vi "Wait for Stream.vi"(5 "timeout in milliseconds":u32=5000, 8 "error in (no error)":errorcluster, 9 "wait for samples transferred":i64=-1, 10 "stream index":i32, 11 "refnum in":refnum<k20>) -> (0 "error out":errorcluster, 1 "samples transferred":u64, 2 "stream state":T1, 3 "refnum out":refnum<k20>)   [LabVIEW 2015, in "niInstr Streaming v1 Host.lvlib"]
doc: "Wait for the specified stream to enter a terminal state (any state that is not Finite or Continuous), or for it to transfer the specified number of samples. If it does not before the timeout is reached, then the VI will throw a timeout error.\n\nSpecifying -1 (the default) for <b>wait for samples transferred</b> shall cause the VI to ignore the number of samples transferred, and only exit on the stream stopping or a timeout.\n\nSpecifying 0 for <b>wait for samples transferred</b> shall cause the VI to immediately return, regardless as to samples transferred. The current number of samples transferred will be reported, as will the stream state.\n\nSpecifying any positive number for <b>wait for samples transferred</b> shall cause the VI to block until that number of samples is reported as transferred, or until the timeout is reached.\n\nThe number of samples transferred is queried after the state, so if the <B>stream state</B> reports \"Done\" - then the samples transferred accurately reflects the terminal state of the stream. However, it is possible for the stream to report that it is still active, but have the number of samples transferred that would indicate completion.\n\nIf the stream enters the Error state, this VI will immediately complete with an error. However, the state and samples transferred outputs remain valid for this. <B>samples transferred</b> reflects the accurate terminal count when the stream entered the Error state. So a user may use this information to clear out the FIFO of the valid samples that remain.\n\n<B>Input Parameters</B>\n\n<B>error in (no error)</B> 'error in' can accept error information wired from VIs previously called. Use this information to decide if any functionality should be bypassed in the event of errors from other VIs.\n\nRight-click the 'error in' control on the front panel and select 'Explain Error' or 'Explain Warning' from the shortcut menu for more information about the error.\n\n<B>stream index</B> Selects which stream index this VI will interface to. This is the index number at the end of the host interface controls (0..7).\n\n<B>refnum in</B> Wire in the session obtained from Open FPGA Reference.\n\n<B>Output Parameters</B>\n\n<B>error out</B> contains error information. This output provides standard error out functionality.\n\n<B>refnum out</B> Copy of refnum in"
uses:
  <instrlib>/_niInstr/Streaming/v1/Host/niInstr Streaming v1 Host.lvlib
  <instrlib>/_niInstr/Streaming/v1/Common/Stream State.ctl
  <instrlib>/_niInstr/Streaming/v1/Host/Public/Stream Host Interface.ctl
  <vilib>/Utility/error.llb/Error Cluster From Error Code.vi
  <vilib>/ErrorRing/Error Ring.xnode
  <instrlib>/_niInstr/Streaming/v1/Common/niInstr Streaming v1 Common.lvlib
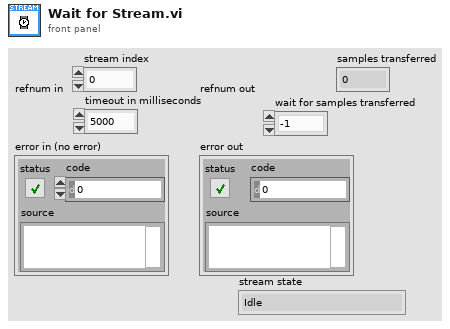
[diagram p1: front panel]
types:
  T1 = typedef "niInstr Streaming v1 Common.lvlib/Stream State.ctl" = enum8{"Idle", "Finite Transfer", "Continuous", "Done", "Error", "Not Ready", "Cancel"}
  T2 = typedef "niInstr Streaming v1 Host.lvlib/Stream Host Interface.ctl" = refnum<k20>
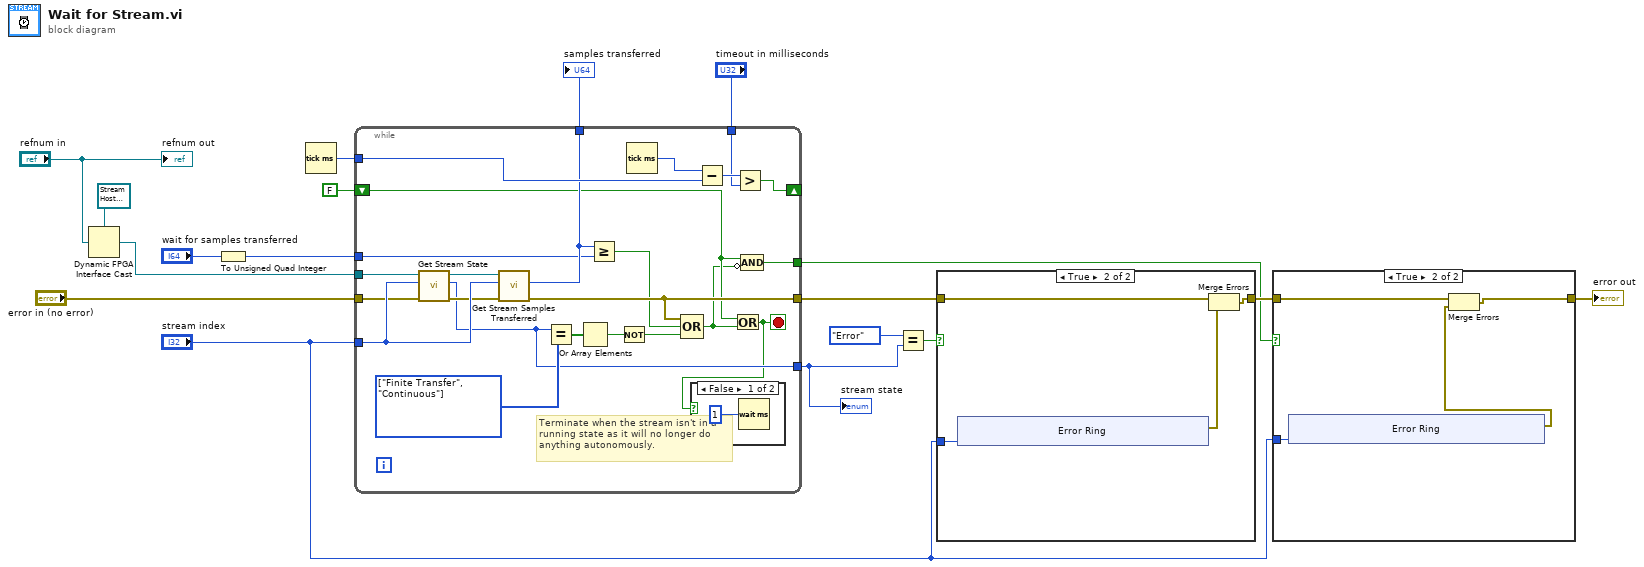
[diagram p0: block diagram]
diagram:
  n1 = Dynamic FPGA Interface Cast(Session In=T2 refnum ("Refnum in"), Type="refnum in") -> (Session Out=w15:T2)
  n2 = To Unsigned Quad Integer(1:"wait for samples transferred") -> (0:w2:u64)
  n3 = Tick Count (ms)() -> (millisecond timer value=w18:u32)
  n4 = while {
    tunnel: w15 -> [w29]
    tunnel: "error in (no error)" -> [w30]
    tunnel: w18 -> [w41]
    tunnel: [w25] -> w6
    tunnel: "stream index" -> [w33]
    tunnel: "timeout in milliseconds" -> [w36]
    tunnel: [w26] -> w10
    tunnel: w2 -> [w31]
    tunnel: [w32] -> w11
    shift-right: [w38] -> _
    shift-left: FALSE -> [w22]
    tunnel: [w23] -> w3
    stop <- w19 stop-if-true
    w34 = T1[] [enum."Finite Transfer", enum."Continuous"] items=["Idle", "Finite Transfer", "Continuous", "Done", "Error", "Not Ready", "Cancel"]
    # "Terminate when the stream isn't in a\nrunning state as it will no longer do\nanything autonomously."
    n5 = call <instrlib>:"Get Stream State.vi"("error in (no error)"=w30, "stream index"=w33, "refnum in"=w29) -> ("error out"=w28:errorcluster, "stream state"=w26:T1, "refnum out"=w27:T2)  [unwired: 6 in]
    n6 = call <instrlib>:"Get Stream Samples Transferred.vi"("error in (no error)"=w28, "stream index"=w33, "refnum in"=w27) -> ("error out"=w25:errorcluster, "samples transferred"=w32:u64)  [unwired: 6 in, 1 out]
    n7 = Equal?(x=w26, y=w34) -> (x = y?=w37:bool[])
    n8 = Or Array Elements(Boolean array=w37) -> (logical OR=w35:bool)
    n9 = Greater Or Equal?(x=w32, y=w31) -> (x >= y?=w20:bool)
    n10 = Not(x=w35) -> (.not. x?=w24:bool)
    n11 = Tick Count (ms)() -> (millisecond timer value=w40:u32)
    n12 = Compound Arithmetic op=OR(w25, w20, w24) -> (w21:bool)
    n13 = Subtract(x=w40, y=w41) -> (x-y=w39:u32)
    n14 = Or(x=w22, y=w21) -> (x .or. y?=w19:bool)
    n15 = case shown="False" w19 {
      frame False {
        n16 = Wait (ms)(milliseconds to wait=u32 1) -> ()  [unwired: 1 out]
      }
      frame True {
      }
    }
    n17 = Greater?(x=w39, y=w36) -> (0:w38:bool)
    n18 = Compound Arithmetic op=AND(w22, invert w21) -> (w23:bool)
  }
  "samples transferred" <- w11
  "stream state" <- w10
  n19 = Equal?(x=Stream_State."Error" ("stream.request state 0"), y=w10) -> (x = y?=w7:bool)
  n20 = case shown="True" w7 {
    tunnel: w6 -> [w43 w47]
    tunnel: [w43 w46] -> w5
    tunnel: "stream index" -> [_ w45]
    frame False {
    }
    frame True {
      n21 = xnode "Error Ring"("parameter 0"=w45) -> ("error out"=w44:errorcluster)
      n22 = Merge Errors(w47, w44) -> (w46:errorcluster)
    }
  }
  n23 = case shown="True" w3 {
    tunnel: w5 -> [w55 w59]
    tunnel: [w55 w58] -> w4
    tunnel: "stream index" -> [_ w56]
    frame False {
    }
    frame True {
      n24 = xnode "Error Ring"("parameter 0"=w56) -> ("error out"=w57:errorcluster)
      n25 = Merge Errors(w59, w57) -> (w58:errorcluster)
    }
  }
  "error out" <- w4
  "refnum out" <- "refnum in"
